vi "SetGenNOsc.vi"(5 "Input Voltage":dbl=1.0, 6 "Amp Scaler":dbl=1.0, 7 "NChannels":i32, 8 "error in (no error)":errorcluster, 9 "Output Voltage":dbl=1.0, 10 "VISA resource name":refnum<visa-resource-name>="Oscilloscope", 11 "AWG VISA":refnum<visa-resource-name>="Generator_1") -> (0 "error out 2":errorcluster)   [LabVIEW 2012]
uses:
  Sum_Abrilader/L0_Sum_Adder Folder/C/Program Files/National Instruments/LabVIEW 2012/instr.lib/Agilent 8000 Series/Agilent 8000 Series.lvlib
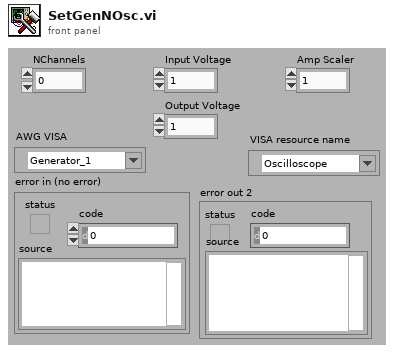
[diagram p1: front panel]
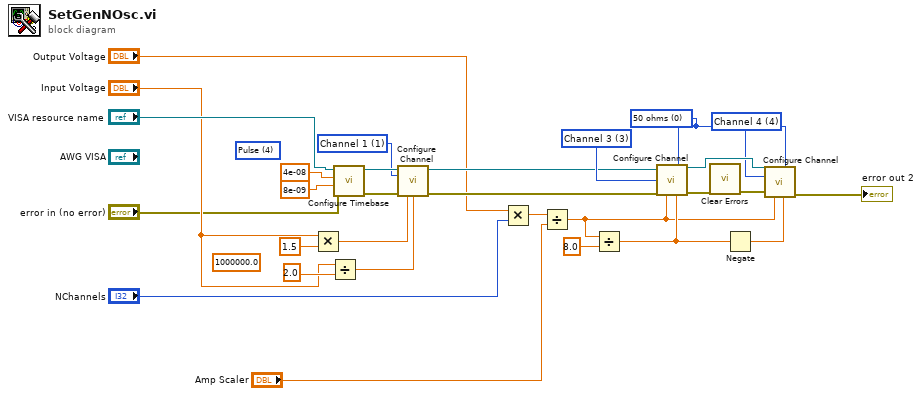
[diagram p0: block diagram]
diagram:
  w17 = u32 0 items=["50 ohms", "1 Mohms"] ("Input Impedance (1: 1 Mohms)")
  w15 = 3 items=["Channel 1"=1, "Channel 2"=2, "Channel 3"=3, "Channel 4"=4] ("Channel (1: Channel 1)")
  w14 = 4 items=["Channel 1"=1, "Channel 2"=2, "Channel 3"=3, "Channel 4"=4] ("Channel (1: Channel 1)")
  w21 = 1 items=["Channel 1"=1, "Channel 2"=2, "Channel 3"=3, "Channel 4"=4] ("Channel (1: Channel 1)")
  (unwired) u16 4 items=["Sine", "Square", "Ramp Up", "Ramp Down", "Pulse", "Noise", "DC"] ("Waveform (0: Sine)")
  (unwired) 1000000.0 ("Frequency (1000.0 Hz)")
  n1 = Multiply(x="Input Voltage", y=1.5) -> (x*y=w25:dbl)
  n2 = Divide(x="Input Voltage", y=2.0) -> (x/y=w22:dbl)
  n3 = call "Configure Timebase.vi"("error in (no error)"="error in (no error)", "Position (0.0 s)"=8e-09, "Timebase (0.005 s)"=4e-08, "VISA resource name"="VISA resource name") -> ("error out"=w29:errorcluster, "VISA resource name out"=w28:refnum<visa-resource-name>)  [unwired: 6 in]
  n4 = call "Configure Channel.vi"("VISA resource name"=w28, "Channel (1: Channel 1)"=w21, "error in (no error)"=w29, "Vertical Range (2.0 V)"=w25, "Vertical Offset (0.0 V)"=w22) -> ("VISA resource name out"=w9:refnum<visa-resource-name>, "error out"=w8:errorcluster)  [unwired: 9 in]
  n5 = Multiply(x="Output Voltage", y="NChannels") -> (x*y=w10:dbl)
  n6 = Divide(x=w10, y="Amp Scaler") -> (x/y=w4:dbl)
  n7 = Divide(x=w4, y=8.0) -> (x/y=w11:dbl)
  n8 = call "Configure Channel.vi"("VISA resource name"=w9, "Input Impedance (1: 1 Mohms)"=w17, "Channel (1: Channel 1)"=w15, "error in (no error)"=w8, "Vertical Range (2.0 V)"=w4, "Vertical Offset (0.0 V)"=w11) -> ("VISA resource name out"=w18:refnum<visa-resource-name>, "error out"=w19:errorcluster)  [unwired: 8 in]
  n9 = call <vilib>:"Clear Errors.vi"("error in (no error)"=w19) -> ("error out"=w16:errorcluster)  [unwired: 6 in]
  n10 = Negate(x=w11) -> (-x=w13:dbl)
  n11 = call "Configure Channel.vi"("VISA resource name"=w18, "Input Impedance (1: 1 Mohms)"=w17, "Channel (1: Channel 1)"=w14, "error in (no error)"=w16, "Vertical Range (2.0 V)"=w4, "Vertical Offset (0.0 V)"=w13) -> ("error out"=→"error out 2":errorcluster)  [unwired: 8 in, 1 out]
